vi "cleanATIData (SubVI).vi"(0 "raw data":dbl[][](array[numeric]), 1 "raw trigger":dbl[][](array[numeric])) -> (2 "raw data":dbl[][](array[numeric]), 4 "stamped data":dbl[][](array[numeric]), 5 "data":waveform(dbl)[](array[waveform]))   [LabVIEW 2017]
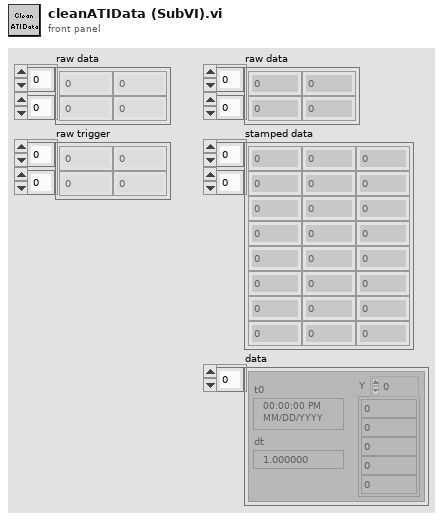
[diagram p1: front panel]
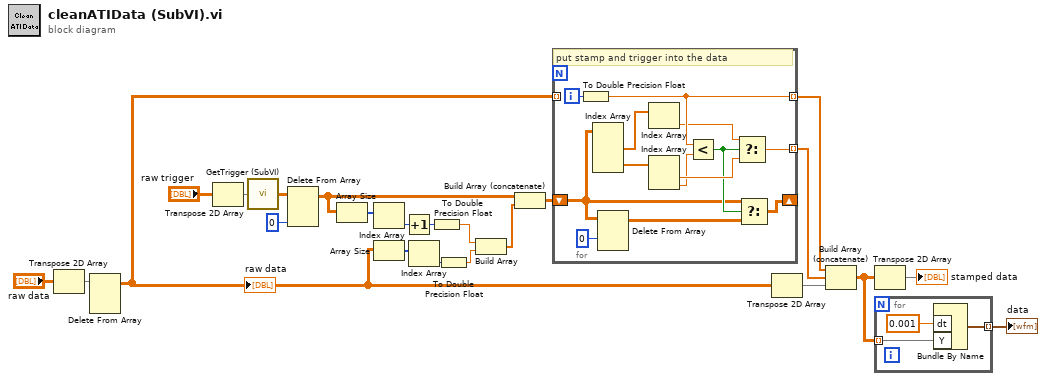
[diagram p0: block diagram]
diagram:
  n1 = Transpose 2D Array(2D array="raw data") -> (transposed array=w21:dbl[][])
  n2 = Delete From Array(array=w21) -> (array with subset deleted=w11:dbl[][])  [unwired: 3 in, 1 out]
  "raw data" <- w11
  n3 = Transpose 2D Array(2D array="raw trigger") -> (transposed array=w22:dbl[][])
  n4 = call "GetTrigger (SubVI).vi"("Array in"=w22) -> ("Array out"=w15:dbl[][])  [unwired: 4 in]
  n5 = Delete From Array(array=w15, index (col)=0 ("disabled index (col)")) -> (array with subset deleted=w6:dbl[][])  [unwired: 2 in, 1 out]
  n6 = Array Size(array=w6) -> (size(s)=w5:i32[])
  n7 = Index Array(array=w5) -> (element=w4:i32)  [unwired: 1 in]
  n8 = Array Size(array=w11) -> (size(s)=w9:i32[])
  n9 = Increment(x=w4) -> (x+1=w3:i32)
  n10 = Index Array(array=w9) -> (element=w10:i32)  [unwired: 1 in]
  n11 = To Double Precision Float(number=w3) -> (double precision float=w2:dbl)
  n12 = To Double Precision Float(number=w10) -> (double precision float=w8:dbl)
  n13 = Build Array(w2, w8) -> (w7:dbl[])
  n14 = Build Array (concatenate)(w6, w7) -> (w12:dbl[][])
  n15 = for {
    tunnel: w11 -> [_] mode=indexing
    tunnel: [w35] -> w23 mode=indexing
    shift-right: [w25] -> _
    shift-left: w12 -> [w27]
    tunnel: [w24] -> w13 mode=indexing
    i -> [w36]
    # "put stamp and trigger into the data"
    n16 = To Double Precision Float(number=w36) -> (double precision float=w35:dbl)
    n17 = Index Array(array=w27) -> (element #1=w33:dbl[], element #2=w31:dbl[])  [unwired: 4 in]
    n18 = Delete From Array(array=w27, index (row)=0 ("index")) -> (array with subset deleted=w26:dbl[][])  [unwired: 2 in, 1 out]
    n19 = Index Array(array=w33) -> (element=w32:dbl)  [unwired: 1 in]
    n20 = Index Array(array=w31) -> (element #1=w30:dbl, element #2=w29:dbl)  [unwired: 2 in]
    n21 = Less?(x=w35, y=w29) -> (x < y?=w28:bool)
    n22 = Select(t=w32, s=w28, f=w30) -> (s? t:f=w24:dbl)
    n23 = Select(t=w27, s=w28, f=w26) -> (s? t:f=w25:dbl[][])
  }
  n24 = Transpose 2D Array(2D array=w11) -> (transposed array=w19:dbl[][])
  n25 = Build Array (concatenate)(w23, w13, w19) -> (w17:dbl[][])
  n26 = Transpose 2D Array(2D array=w17) -> (transposed array=→"stamped data":dbl[][])
  n27 = for {
    tunnel: w17 -> [w39] mode=indexing
    tunnel: [w37] -> w18 mode=indexing
    n28 = Bundle By Name("dt"=0.001, "Y"=w39) -> (w37:waveform(dbl))  [unwired: 1 in]
  }
  "data" <- w18
